vi "VI Linearisierung v2.vi"() -> ()   [LabVIEW 2020, in "Linearisierung v2.lvlib"] (continued)
      n463 = Select(t=T66."Disabled and Grayed Out" ("Deaktiviert"), s=w534, f=w533) -> (s? t:f=w550:T66)
      n464 = Select(t=FALSE ("x = y?"), s=w534, f=w552) -> (s? t:f=w554:T1)
      n465 = Select(t=u16 0, s=w534, f=w543) -> (s? t:f=w555:u16)
      n466 = Select(t=T66."Disabled and Grayed Out" ("Deaktiviert"), s=w535, f=w533) -> (s? t:f=w532:T66)
      n467 = property on="Gasteilerkorrektur" class="Bool."("Visible"=w534) -> (error out=w576:errorcluster)  [unwired: 2 in, 1 out]
      n468 = property on="Registerkarte" class="RKElem (strikt)"("Visible"=w574) -> (error out=w581:errorcluster)  [unwired: 2 in, 1 out]
      n469 = property on="Error" class="Cluster (strikt)"("Visible"=w574) -> (error out=w582:errorcluster)  [unwired: 2 in, 1 out]
      n470 = property on="Störung Kommunikation" class="Bool. (strikt)"("Visible"=w574) -> (error out=w583:errorcluster)  [unwired: 2 in, 1 out]
      n471 = property on="TCP Verbindung aktiv" class="Bool. (strikt)"("Visible"=w574) -> (error out=w584:errorcluster)  [unwired: 2 in, 1 out]
      n472 = property on="Error" class="Cluster (strikt)"("Visible"=w574) -> (error out=w578:errorcluster)  [unwired: 2 in, 1 out]
      n473 = property on="Anforderung" class="Bool. (strikt)"("Visible"=w574) -> (error out=w577:errorcluster)  [unwired: 2 in, 1 out]
      n474 = property on="ABBRECHEN" class="Bool."("Visible"=w574) -> (error out=w573:errorcluster)  [unwired: 2 in, 1 out]
      n475 = property on="STARTEN" class="Bool. (strikt)"("Visible"=w574) -> (error out=w572:errorcluster)  [unwired: 2 in, 1 out]
      n476 = property on="automatisch" class="Bool. (strikt)"("DisabledEnum"=w550, "Value"=w554) -> (error out=w558:errorcluster)  [unwired: 2 in, 1 out]
      n477 = property on="Gasteiler Span Eingänge" class="Ring (strikt)"("DisabledEnum"=w532, "Value"=w555, "Visible"=w519) -> (error out=w557:errorcluster)  [unwired: 2 in, 1 out]
      n478 = control-ref of="Eingabetabelle"() -> (w559:refnum<vi>)
      n479 = control-ref of="Ausgabetabelle"() -> (w542:refnum<vi>)
      n480 = control-ref of="EPA Ausgabetabelle"() -> (w563:refnum<vi>)
      n481 = control-ref of="LIN Ausgabetabelle"() -> (w562:refnum<vi>)
      n482 = local write "Gasteilerstatus"("" ("Gasteilerstatus")) -> ()
      n483 = call <vilib>:"Clear Errors.vi"("error in (no error)"=w596) -> ("error out"=w595:errorcluster)  [unwired: 5 in, 1 out]
      n484 = call "Einheiten finden.vi"("Komponente"=w568) -> ("Einheit in String"=w561:string)  [unwired: 6 in, 4 out]
      n485 = control-ref of="PDF single pages Components"() -> (w524:refnum<vi>)
      n486 = control-ref of="PDF single pages Span"() -> (w523:refnum<vi>)
      n487 = control-ref of="PDF Deckblatt"() -> (w522:refnum<vi>)
      n488 = control-ref of="PDF öffnen"() -> (w521:refnum<vi>)
      n489 = call "Einheiten in Tabellenspalten.vi"("Einheit"=w561, "Tabelle (Eingang)"=w559) -> ("Einheit out"=w560:string)  [unwired: 7 in, 2 out]
      n490 = local write "Einheit"(w561) -> ()
      n491 = local write "Einheit Deviation"(w561) -> ()
      n492 = call "Einheiten in Tabellenspalten.vi"("Einheit"=w560, "Tabelle (Eingang)"=w542) -> ("error out"=w567:errorcluster, "Einheit out"=w565:string)  [unwired: 7 in, 1 out]
      n493 = Bundle("PDF single pages Components"=w524, "PDF single pages Span"=w523, "PDF Deckblatt"=w522, "PDF öffnen"=w521) -> (w520:T130)  [unwired: 1 in]
      n494 = call "Einheiten in Tabellenspalten.vi"("error in (no error)"=w567, "Einheit"=w565, "Tabelle (Eingang)"=w563) -> ("error out"=w566:errorcluster, "Einheit out"=w564:string)  [unwired: 6 in, 1 out]
      n495 = Merge Errors(w576, w581, w582, w583, w584, w578, w577, w573, w572, w558, w557) -> (w580:errorcluster)
      n496 = call "GD_MG_MagicFormula_OnOff.vi"("Aktion"=enum16{"lesen", "schreiben", "init"}."init") -> ()  [unwired: 8 in, 2 out]
      n497 = call "Einheiten in Tabellenspalten.vi"("error in (no error)"=w566, "Einheit"=w564, "Tabelle (Eingang)"=w562) -> ()  [unwired: 6 in, 3 out]
      n498 = call <vilib>:"Clear Errors.vi"("error in (no error)"=w580) -> ()  [unwired: 5 in, 2 out]
    }
    frame #5 {
      # "#LIN_Hakerl"
      n499 = local read "TCP Verbindung aktiv"() -> (w668:bool)
      n500 = call "FGV CalGas.vi"("Aktionen"=FGV_CalGas_Aktionen."KAL extrahieren") -> ("Aufschaltung CalGas"=w650:T131)  [unwired: 6 in, 4 out]
      n501 = local write "Aufschaltung CalGas"(w650) -> ()
      n502 = Boolean To (0,1)(Boolean=w668) -> (0, 1=w667:i16)
      n503 = local write "Registerkarte"(w667) -> ()
      n504 = property on="FORTSETZEN" class="Bool."("Visible"=FALSE ("Sichtbar")) -> (error out=w653:errorcluster)  [unwired: 2 in, 1 out]
      n505 = call <vilib>:"Clear Errors.vi"("error in (no error)"=w653) -> ()  [unwired: 5 in, 2 out]
      n506 = call "Tabelle in die einzelnen Seiten zerlegen.vi"("Aktion"=FGV_Aktion_Tabelle_zerlegen."vereinzeln", "Index (Seite)"=41) -> ("Sprachliste"=w655:string[][])  [unwired: 7 in, 2 out]
      n507 = call "FGV Gasliste.vi"("Aktionen"=FGV_FT-IR_Gasliste_Aktionen."lesen") -> ("Aktuelle Gasliste gesamt"=w652:T48[])  [unwired: 8 in, 2 out]
      n508 = call "Tabelle in die einzelnen Seiten zerlegen.vi"("Aktion"=FGV_Aktion_Tabelle_zerlegen."vereinzeln", "Index (Seite)"=35) -> ("Sprachliste"=w661:string[][])  [unwired: 7 in, 2 out]
      n509 = call "Texte in VIs uebersetzen.vi"("Sprachliste"=w661, "String-Array zum Übersetzen"=w652, "String zum Übersetzen"="Temp. Messzelle" ("Neues Element/Teil-Array")) -> ("String-Array zum Übersetzen"=w659:string[], "String zum Übersetzen"=w663:string)  [unwired: 8 in, 3 out]
      n510 = call "String in Array suchen.vi"("Nach String/Zeichen suchen (-)"=w663, "String-Array"=w659) -> ("Index"=w665:i32)  [unwired: 7 in, 2 out]
      n511 = control-ref of="ABBRECHEN"() -> (w649:refnum<vi>)
      n512 = call "Texte in VIs uebersetzen.vi"("Sprachliste"=w655, "String zum Übersetzen"="Kalibrierung:" ("Status kalibrieren")) -> ("String zum Übersetzen"=w656:string)  [unwired: 9 in, 4 out]
      n513 = control-ref of="Ergebnis PDF TRUE"() -> (w643:refnum<vi>)
      n514 = control-ref of="Ergebnis PDF FALSE"() -> (w642:refnum<vi>)
      n515 = local write "Status kalibrieren"(w656) -> ()
      n516 = property class="Bool."(reference=w649, "DisabledEnum"=T66."Disabled and Grayed Out" ("Deaktiviert")) -> (reference out=w648:refnum<vi>, error out=w646:errorcluster)  [unwired: 1 in]
      n517 = Bundle By Name(cluster=T97 {"Yes Ctl Refnum"=refnum, "No Ctl Refnum"=refnum} ("ResultPictures"), "Yes Ctl Refnum"=w643, "No Ctl Refnum"=w642) -> (w641:T97)
      n518 = call <vilib>:"Clear Errors.vi"("error in (no error)"=w646) -> ()  [unwired: 5 in, 2 out]
      n519 = control-ref of="STARTEN"() -> (w645:refnum<vi>)
      "Ergebnis PDF TRUE" <- T3 TRUE ("Ergebnis PDF TRUE")
      "Ergebnis PDF FALSE" <- T3 FALSE ("Ergebnis PDF FALSE")
    }
    frame #6 {
      # "War der GD ein Horiba GDC und das VI wurde\ngestoppt, stimmen beim Start die Error Flags nicht ...."
      n520 = local read "Gasteiler Type"() -> (w671:T15)
      n521 = property on="Gasteiler Type" class="Ring (strikt)"("Val(Sgnl)"=w671) -> (error out=w670:errorcluster)  [unwired: 2 in, 1 out]
      n522 = call <vilib>:"Clear Errors.vi"("error in (no error)"=w670) -> ()  [unwired: 5 in, 2 out]
    }
    frame #7 {
      n523 = Wait Until Next ms Multiple(millisecond multiple=u32 200 ("ms")) -> (millisecond timer value=w672:u32)
      n524 = flat-sequence {
        tunnel: w672 -> [_]
        frame #0 {
          n525 = call "Spantabellenanzeige.vi"() -> ("SpanTabelle"=w676:T48[][])  [unwired: 10 in, 1 out]
          n526 = Delete From Array(array=w676, length=3 ("Länge"), index (col)=0 ("Deaktivierter Index (Spalte)")) -> (deleted portion=→"SpanTabelleAnzeige":T48[][], array with subset deleted=w677:T48[][])  [unwired: 1 in]
          n527 = local write "SpanTabelleEingabe"(w677) -> ()
        }
      }
    }
    frame #8 {
      w683 = T4 FALSE  # Gasteiler Spülen
      n528 = call "FT-IR EVID-Codes External Data.vi"("Aktionen"=Aktionen_EVID-Codes."lesen") -> ("Anzahl"=w698:i32)  [unwired: 9 in, 5 out]
      n529 = call "FGV Gasliste.vi"("Aktionen"=FGV_FT-IR_Gasliste_Aktionen."lesen") -> ("Aktuelle Gasliste gesamt"=w689:T48[], "Aktuelle Gasliste FT-IR"=w696:T48[])  [unwired: 8 in, 1 out]
      n530 = call "FGV Span.vi"("Aktion"=Aktion_FGV_Span."Seite aktiv", "Aktiv"=FALSE) -> ()  [unwired: 6 in, 4 out]
      n531 = Add(x=w698, y=3) -> (x+y=w688:i32)
      n532 = control-ref of="SpanTabelleEingabe"() -> (w681:refnum<vi>)
      n533 = Array Size(array=w696) -> (size(s)=w695:i32)
      n534 = Array Size(array=w689) -> (size(s)=w690:i32)
      n535 = control-ref of="PolynomTabelleAnzeige"() -> (w679:refnum<vi>)
      n536 = control-ref of="PolynomTabelleEingabe"() -> (w680:refnum<vi>)
      n537 = disable-structure shown="Deaktiviert" {
        disable-tunnel: w680 -> [w703 _]
        frame Disabled {
          n538 = for {
            N: 5 -> [_]
            tunnel: w703 -> [w707]
            tunnel: T100 {"Row"=0, "Column"=0} ("Aktive Zelle:Aktive Zelle") -> [w706]
            i -> [w705]
            n539 = for {
              N: 200 -> [_]
              tunnel: w707 -> [w714]
              tunnel: w706 -> [w713]
              tunnel: w705 -> [w711]
              i -> [w710]
              n540 = Bundle By Name(cluster=w713, "Column"=w711, "Row"=w710) -> (w712:T100)
              n541 = property class="Tbl (strikt)"(reference=w714, "Active Cell"=w712) -> (reference out=w709:refnum<vi>)  [unwired: 1 in, 1 out]
              n542 = property class="Tbl (strikt)"(reference=w709, "Justify"=enum16{"Left", "Center", "Right"}."Left" ("Aktive Zelle:Zellenausrichtung")) -> ()  [unwired: 1 in, 2 out]
            }
          }
        }
        frame Enabled {
        }
      }
      n543 = Subtract(x=w695, y=w688) -> (x-y=w694:i32)
      n544 = Subtract(x=w690, y=w688) -> (x-y=w687:i32)
      n545 = control-ref of="SpanTabelleAnzeige"() -> (w682:refnum<vi>)
      n546 = call "Zeile faerben.vi"("Anzahl"=w694, "Table (Eingang)"=w682) -> ("error out"=w693:errorcluster)  [unwired: 9 in]
      n547 = call "Zeile faerben.vi"("error in (no error)"=w693, "Anzahl"=w694, "Table (Eingang)"=w681) -> ("error out"=w692:errorcluster)  [unwired: 8 in]
      n548 = call "Zeile faerben.vi"("error in (no error)"=w692, "Anzahl"=w687, "Table (Eingang)"=w680) -> ("error out"=w691:errorcluster)  [unwired: 8 in]
      n549 = call "Zeile faerben.vi"("error in (no error)"=w691, "Anzahl"=w687, "Table (Eingang)"=w679) -> ()  [unwired: 8 in, 1 out]
      n550 = disable-structure shown="TestRun==TRUE" {
        disable-tunnel: [w715 w716] -> w684
        frame condition #0 (active) {
          w715 = TRUE  # TestRun
          # "#TestRun"
        }
        frame condition #1 {
          w716 = FALSE  # TestRun
        }
      }
    }
  }
  n551 = while {
    tunnel: w39 -> [w760]
    tunnel: w37 -> [_]
    shift-right: [w758] -> _
    shift-left: w17 -> [w757]
    shift-right: [w756] -> _
    shift-left: _ -> [w755]
    shift-right: [w754] -> _
    shift-left: _ -> [w753]
    tunnel: w36 -> [w752]
    tunnel: w35 -> [w751]
    tunnel: w34 -> [w750]
    tunnel: w33 -> [w749]
    tunnel: w32 -> [w748]
    tunnel: w31 -> [w747]
    tunnel: w30 -> [w746]
    tunnel: w29 -> [w745]
    tunnel: w28 -> [w744]
    tunnel: w25 -> [w743]
    tunnel: w26 -> [w742]
    tunnel: w27 -> [w741]
    tunnel: w24 -> [w740]
    tunnel: w23 -> [w739]
    tunnel: w19 -> [w738]
    tunnel: w20 -> [w737]
    tunnel: w21 -> [w736]
    tunnel: w22 -> [w735]
    tunnel: w18 -> [w734]
    tunnel: w16 -> [w733]
    tunnel: w15 -> [w732]
    tunnel: w14 -> [w731]
    tunnel: w13 -> [w730]
    tunnel: w12 -> [w729]
    shift-right: [w728] -> _
    shift-left: w38 -> [w759]
    tunnel: w11 -> [w727]
    tunnel: w10 -> [w726]
    tunnel: w9 -> [w725]
    tunnel: w8 -> [w724]
    tunnel: w7 -> [w723]
    tunnel: w6 -> [w722]
    tunnel: w5 -> [w721]
    tunnel: w4 -> [w720]
    tunnel: w3 -> [w718]
    tunnel: w2 -> [w719]
    tunnel: w1 -> [w717]
    stop <- FALSE stop-if-true
    # "250 für Timer"
    n552 = event shown="[26] \"EPA PDF erzeugen\": Wertänderung" {
      selector: _ -> [_ _ _ _ _ _ _ _ _ _ _ _ _ _ _ _ _ _ _ _ _ _ _ _ _ _ _ _ _ _ _ _ _ _ _ _ _ _ _ _ _ _ _ _ _ _ _ _ _ _ _ _ _ _ _ _ _ _ _ _ _]
      dyn-events: _ -> [_ _ _ _ _ _ _ _ _ _ _ _ _ _ _ _ _ _ _ _ _ _ _ _ _ _ _ _ _ _ _ _ _ _ _ _ _ _ _ _ _ _ _ _ _ _ _ _ _ _ _ _ _ _ _ _ _ _ _ _ _]
      timeout: 250 -> [_ _ _ _ _ _ _ _ _ _ _ _ _ _ _ _ _ _ _ _ _ _ _ _ _ _ _ _ _ _ _ _ _ _ _ _ _ _ _ _ _ _ _ _ _ _ _ _ _ _ _ _ _ _ _ _ _ _ _ _ _]
      tunnel: w760 -> [w768 _ _ _ _ _ _ _ _ _ _ _ _ _ _ w1488 w1532 w1567 _ _ w1742 w1765 w1809 _ _ w2079 w2473 _ _ _ _ _ w2652 _ w2893 w2999 w3024 _ w3060 _ _ _ w3174 _ w3242 _ _ _ _ _ _ _ _ _ _ _ _ _ _ _ _]
      tunnel: w759 -> [w796 w1237 w1243 _ w1316 w1333 w1360 w1372 w1388 w1400 w1412 w1430 w1442 w1446 w1459 w1485 w1514 w1565 w1717 w1722 w1739 w1762 w1806 w1844 w1863 w2064 w2479 w2505 w2514 w2521 w2580 w2605 w2628 w2842 w2892 w3000 w3023 w3043 w3057 w3120 w3128 w3148 w3179 w3210 w3244 w3481 w3574 w3584 w3620 w3759 w3812 w3848 w3864 w3888 w4033 w4111 w4115 w4140 w4180 w4341 w4372]
      tunnel: [w810 w1239 w1245 w1278 w1325 w1339 w1364 w1380 w1392 w1404 w1421 w1434 w1445 w1458 w1467 w1491 w1533 w1573 w1721 w1724 w1741 w1764 w1808 w1850 w1872 w2086 w2481 w2507 w2516 w2535 w2587 w2609 w2653 w2857 w2896 w3002 w3033 w3046 w3059 w3127 w3134 w3150 w3198 w3220 w3253 w3494 w3579 w3590 w3650 w3785 w3841 w3863 w3872 w3932 w4080 w4114 w4121 w4143 w4231 w4356 w4374] -> w758
      tunnel: w757 -> [w811 w1239 w1245 w1278 w1325 w1339 w1364 w1380 w1392 w1404 w1421 w1434 w1445 w1458 w1467 w1491 w1533 w1573 w1721 _ w1741 w1764 w1808 w1850 w1872 w2086 w2481 w2507 w2516 w2535 w2587 w2609 w2653 w2857 w2896 w3002 w3033 w3046 w3059 w3127 w3134 w3150 w3198 w3220 w3253 w3494 w3579 w3590 w3650 w3785 w3841 w3863 w3872 w3932 w4080 w4114 w4121 w4143 w4231 w4356 w4374]
      tunnel: [w807 w1238 w1244 w1277 w1324 w1338 w1363 w1379 w1391 w1403 w1420 w1433 w1444 w1457 w1466 w1486 w1531 w1566 w1718 w1723 w1740 w1763 w1807 w1846 w1871 w2085 w2480 w2506 w2515 w2534 w2583 w2608 w2649 w2846 w2895 w3001 w3032 w3045 w3058 w3125 w3133 w3149 w3197 w3219 w3251 w3493 w3578 w3589 w3649 w3784 w3840 w3862 w3871 w3928 w4079 w4112 w4120 w4142 w4230 w4355 w4373] -> w756
      tunnel: w755 -> [w808 w1238 w1244 w1277 w1324 w1338 w1363 w1379 w1391 w1403 w1420 w1433 w1444 w1457 w1466 w1486 w1531 w1566 w1718 w1723 w1740 w1763 w1807 w1846 w1871 w2085 w2480 w2506 w2515 w2534 w2583 w2608 w2649 w2846 w2895 w3001 w3032 w3045 w3058 w3125 w3133 w3149 w3197 w3219 w3251 w3493 w3578 w3589 w3649 w3784 w3840 w3862 w3871 w3928 w4079 w4112 w4120 w4142 w4230 w4355 w4373]
      tunnel: [w806 _ _ _ _ _ _ _ _ _ _ _ _ _ _ _ _ _ _ _ _ _ _ _ _ _ _ _ _ _ _ _ _ _ _ _ _ _ _ _ _ _ _ _ _ _ _ _ _ _ _ _ _ _ _ _ _ _ _ _ _] -> w754
      tunnel: w753 -> [w805 _ _ _ _ _ _ _ _ _ _ _ _ _ _ _ _ _ _ _ _ _ _ _ _ _ _ _ _ _ _ _ _ _ _ _ _ _ _ _ _ _ _ _ _ _ _ _ _ _ _ _ _ _ _ _ _ _ _ _ _]
      tunnel: w752 -> [_ _ _ _ w1323 w1337 w1361 w1378 w1389 w1401 w1419 w1431 _ _ _ _ _ _ _ _ _ _ _ _ _ _ _ _ _ _ _ _ _ _ _ _ _ _ _ _ _ _ _ _ _ _ _ _ _ _ _ _ _ _ _ _ _ _ _ _ _]
      tunnel: w751 -> [_ _ _ _ _ _ _ _ _ _ _ _ _ _ _ _ _ _ _ _ _ _ _ _ _ _ _ _ _ _ _ _ _ _ _ _ _ _ _ _ _ _ _ _ _ _ _ _ _ _ _ _ _ _ w4065 _ _ _ _ _ _]
      tunnel: w750 -> [_ _ _ _ _ _ _ _ _ _ _ _ _ _ _ _ _ _ _ _ _ _ _ _ _ _ _ _ _ _ _ _ w2638 _ _ _ _ _ _ _ _ _ w3190 _ w3238 w3484 _ _ _ _ _ _ _ w3899 _ _ _ _ _ _ _]
      tunnel: w749 -> [_ _ _ _ _ _ _ _ _ _ _ _ _ _ _ _ _ _ _ _ _ _ _ _ _ _ _ _ _ _ _ _ w2635 _ _ _ _ _ _ _ _ _ w3187 _ w3233 _ _ _ _ _ _ _ _ _ _ _ _ _ _ _ _]
      tunnel: w748 -> [_ _ _ _ _ _ _ _ _ _ _ _ _ _ _ _ _ _ _ _ _ _ _ _ _ _ _ _ _ _ _ _ _ _ _ _ _ _ _ _ _ _ w3196 _ _ _ _ _ _ _ _ _ _ _ _ _ _ _ _ _ _]
      tunnel: w747 -> [_ _ _ _ _ _ _ _ _ _ _ _ _ _ _ _ _ _ _ _ _ _ _ _ _ _ _ _ _ _ _ _ w2637 _ _ _ _ _ _ _ _ _ w3189 _ w3235 _ _ _ _ _ _ _ _ _ _ _ _ _ _ _ _]
      tunnel: w746 -> [_ _ _ _ _ _ _ _ _ _ _ _ _ _ _ _ _ _ _ _ _ _ _ _ _ _ _ _ _ _ _ _ w2636 _ _ _ _ _ _ _ _ _ w3188 _ w3234 w3489 _ _ _ _ _ _ _ w3902 _ _ _ _ _ _ _]
      tunnel: w745 -> [w775 _ _ _ _ _ _ _ _ _ _ _ _ _ _ _ _ _ _ _ _ _ _ _ _ w2078 w2478 _ _ _ _ _ w2645 w2843 _ _ _ _ _ w3122 _ _ _ _ _ _ _ _ _ _ _ _ _ _ _ _ _ _ _ _ _]
      tunnel: w744 -> [w782 _ _ _ _ _ _ _ _ _ _ _ _ _ _ _ _ _ _ _ _ _ _ _ _ _ _ _ _ _ _ _ w2642 _ _ _ _ _ _ _ _ _ _ _ _ _ _ _ _ _ _ _ _ _ _ _ _ _ _ _ _]
      tunnel: w743 -> [_ _ _ _ _ _ _ _ _ _ _ _ _ _ _ _ _ _ _ _ _ _ _ _ w1868 _ _ _ _ _ _ _ w2632 _ _ _ _ _ _ _ _ _ w3185 _ w3229 w3452 _ _ w3646 _ _ w3849 _ _ _ _ _ _ _ _ _]
      tunnel: w742 -> [_ _ _ _ _ _ _ _ _ _ _ _ _ _ _ _ _ _ _ _ _ _ _ _ w1866 _ _ _ _ _ _ _ _ _ _ _ _ _ _ _ _ _ _ _ _ _ _ _ w3644 _ _ _ _ _ _ _ _ _ _ _ _]
      tunnel: w741 -> [_ _ _ _ _ _ _ _ _ _ _ _ _ _ _ _ _ _ _ _ _ _ _ _ w1867 _ _ _ _ _ _ _ _ _ _ _ _ _ _ _ _ _ _ _ _ _ _ _ w3645 _ _ _ _ _ _ _ _ _ _ _ _]
      tunnel: w740 -> [_ _ _ _ _ _ _ _ _ _ _ _ _ _ _ _ _ _ _ _ _ _ _ _ _ _ _ _ _ _ _ _ w2634 _ _ _ _ _ _ _ _ _ w3186 _ w3230 w3453 _ _ w3643 _ _ w3850 _ _ _ _ _ _ _ _ _]
      tunnel: w739 -> [_ _ _ _ _ _ _ _ _ _ _ _ _ _ _ _ _ _ _ _ _ _ _ _ _ _ _ _ _ _ _ _ _ _ _ _ _ _ _ _ _ _ _ _ _ _ _ _ _ _ _ _ _ _ w4034 _ _ _ _ _ _]
      tunnel: w738 -> [_ _ _ _ _ _ _ _ _ _ _ _ _ _ _ _ _ _ _ _ _ _ _ _ _ _ _ _ _ _ _ _ _ _ _ _ _ _ _ _ _ _ _ _ _ _ _ _ _ _ _ _ _ _ _ _ _ _ w4192 _ _]
      tunnel: w737 -> [_ _ _ _ _ _ _ _ _ _ _ _ _ _ _ _ _ _ _ _ _ _ _ _ _ _ _ _ _ _ _ _ _ _ _ _ _ _ _ _ _ _ _ _ _ _ _ _ _ _ _ _ _ _ _ _ _ _ w4191 _ _]
      tunnel: w736 -> [w798 _ _ _ _ _ _ _ _ _ _ _ _ _ _ _ _ _ _ _ _ _ _ _ w1861 _ _ _ _ _ _ _ _ _ _ _ _ _ _ _ _ _ _ _ _ _ _ _ _ _ _ _ _ _ _ _ _ _ w4184 w4348 _]
      tunnel: w735 -> [w797 _ _ _ _ _ _ _ _ _ _ _ _ _ _ _ _ _ _ _ _ _ _ _ w1862 _ _ _ _ _ _ _ _ _ _ _ _ _ _ _ _ _ _ _ _ _ _ _ _ _ _ _ _ _ _ _ _ _ w4183 w4347 _]
      tunnel: w734 -> [_ _ _ _ _ _ _ _ _ _ _ _ _ _ _ _ _ _ _ _ _ _ _ _ _ _ _ _ _ _ _ _ w2627 _ _ _ _ _ _ _ _ _ w3171 _ w3231 _ _ _ _ _ _ _ w3870 _ _ _ _ _ _ _ _]
      tunnel: w733 -> [w776 _ _ _ _ _ _ _ _ _ _ _ _ _ _ _ _ _ _ _ _ _ _ _ _ _ _ _ _ _ _ _ _ _ _ _ _ _ _ _ _ _ _ _ _ _ _ _ _ _ _ _ _ _ _ _ _ _ _ _ _]
      tunnel: w732 -> [_ _ _ w1276 _ _ _ _ _ _ _ _ _ _ _ _ _ _ _ _ _ _ _ _ _ _ _ _ _ _ _ _ _ _ _ _ _ _ _ _ _ _ _ _ _ _ _ _ _ _ _ _ _ _ _ _ _ _ _ _ _]
      tunnel: w731 -> [_ _ _ w1275 _ _ _ _ _ _ _ _ _ _ _ _ _ _ _ _ _ _ _ _ _ _ _ _ _ _ _ _ _ _ _ _ _ _ _ _ _ _ _ _ _ _ _ _ _ _ _ _ _ _ _ _ _ _ _ _ _]
      tunnel: w730 -> [_ _ _ w1274 _ _ _ _ _ _ _ _ _ _ _ _ _ _ _ _ _ _ _ _ _ _ _ _ _ _ _ _ _ _ _ _ _ _ _ _ _ _ _ _ _ _ _ _ _ _ _ _ _ _ _ _ _ _ _ _ _]
      tunnel: w729 -> [_ _ _ w1273 _ _ _ _ _ _ _ _ _ _ _ _ _ _ _ _ _ _ _ _ _ _ _ _ _ _ _ _ _ _ _ _ _ _ _ _ _ _ _ _ _ _ _ _ _ _ _ _ _ _ _ _ _ _ _ _ _]
      tunnel: [w796 w1237 w1243 w1272 w1316 w1333 w1360 w1372 w1388 w1400 w1412 w1430 w1442 w1446 w1459 w1485 w1514 w1565 w1717 w1722 w1739 w1762 w1806 w1844 w1863 w2064 w2479 w2505 w2514 w2521 w2580 w2605 w2628 w2842 w2892 w3000 w3023 w3043 w3057 w3120 w3128 w3148 w3179 w3210 w3244 w3481 w3574 w3584 w3620 w3759 w3812 w3848 w3864 w3888 w4033 w4111 w4115 w4140 w4180 w4341 w4372] -> w728
      tunnel: w727 -> [_ _ w1242 _ _ _ _ _ _ _ _ _ _ _ _ _ _ _ _ _ _ _ _ _ _ _ _ _ _ _ _ _ _ _ _ _ _ _ _ _ _ _ _ _ _ _ _ _ _ _ _ _ _ _ _ _ _ _ _ _ _]
      tunnel: w726 -> [_ _ w1241 _ _ _ _ _ _ _ _ _ _ _ _ _ _ _ _ _ _ _ _ _ _ _ _ _ _ _ _ _ _ _ _ _ _ _ _ _ _ _ _ _ _ _ _ _ _ _ _ _ _ _ _ _ _ _ _ _ _]
      tunnel: w725 -> [_ _ w1240 _ _ _ _ _ _ _ _ _ _ _ _ _ _ _ _ _ _ _ _ _ _ _ _ _ _ _ _ _ _ _ _ _ _ _ _ _ _ _ _ _ _ _ _ _ _ _ _ _ _ _ _ _ _ _ _ _ _]
      tunnel: w724 -> [_ _ _ _ _ _ _ _ _ _ _ _ _ _ _ _ _ _ _ _ _ _ _ _ _ w2059 _ _ _ _ _ _ _ _ _ _ _ _ _ _ _ _ _ _ _ _ _ _ _ _ _ _ _ _ _ _ _ _ _ _ _]
      tunnel: w723 -> [_ _ _ _ _ _ _ _ _ _ _ _ _ _ _ _ _ _ _ _ _ _ _ _ _ w2056 w2475 _ _ _ _ _ _ _ _ _ _ _ _ _ _ _ _ _ _ _ _ _ _ _ _ _ _ _ _ _ _ _ _ _ _]
      tunnel: w722 -> [_ _ _ _ _ _ _ _ _ _ _ _ _ _ _ _ _ _ _ _ _ _ _ _ _ w2055 w2476 _ _ _ _ _ _ _ _ _ _ _ _ _ _ _ _ _ _ _ _ _ _ _ _ _ _ _ _ _ _ _ _ _ _]
      tunnel: w721 -> [_ _ _ _ _ _ _ _ _ _ _ _ _ _ _ _ _ _ _ _ _ _ _ _ _ w2054 w2477 _ _ _ _ _ _ _ _ _ _ _ _ _ _ _ _ _ _ _ _ _ _ _ _ _ _ _ _ _ _ _ _ _ _]
      tunnel: w720 -> [_ _ _ _ _ _ _ _ _ _ _ _ _ _ _ _ _ _ _ _ _ _ _ _ _ w2049 w2474 _ _ _ _ _ _ _ _ _ _ _ _ _ _ _ _ _ _ _ _ _ _ _ _ _ _ _ _ _ _ _ _ _ _]
      tunnel: w718 -> [_ _ _ _ _ _ _ _ _ _ _ _ _ _ _ _ _ _ _ _ _ _ _ _ _ w2047 _ w2499 _ _ _ _ _ _ _ _ _ _ _ _ _ _ _ _ _ _ _ _ w3611 _ _ _ _ _ _ _ _ _ _ _ _]
      tunnel: w719 -> [_ _ _ _ _ _ _ _ _ _ _ _ _ _ _ _ _ _ _ _ _ _ _ _ _ _ _ _ _ _ _ _ _ _ _ _ _ _ _ _ _ _ w3168 _ w3227 w3436 _ _ _ _ _ _ _ _ _ _ _ _ _ _ _]
      tunnel: w717 -> [_ _ _ _ _ _ _ _ _ _ _ _ _ _ _ _ _ _ _ _ _ _ _ _ _ _ _ w2500 w2513 _ _ _ _ _ _ _ _ _ _ _ _ _ _ _ _ _ _ _ w3610 _ _ _ _ _ _ _ _ _ _ _ _]
      event Timeout {
        w769 = TRUE  # get Test Data
        n553 = event-data() -> ("Source"=w784:T158, "Type"=w786:T159, "Time"=w785:u32)  [unwired: 1 in]
        n554 = control-ref of="FORTSETZEN"() -> (w774:refnum<vi>)
        n555 = control-ref of="Speichern LIN"() -> (w773:refnum<vi>)
        n556 = call "GD_MG_MagicFormula_OnOff.vi"("Aktion"=enum16{"lesen", "schreiben", "init"}."lesen") -> ("use old LNI"=w787:bool, "MG_use_magic_formula"=w788:bool)  [unwired: 8 in]
        n557 = local read "Hauptregisterkarte"() -> (w813:T8)
        n558 = call "Komponentenausgabe.vi"() -> ("Gaskomponente"=w814:T7)  [unwired: 8 in, 3 out]
        n559 = call "FGV Daten Abholung uebergeben.vi"("Aktion"=Aktion_FGV_Daten_Abholung_uebergebenctl."lesen") -> ("Zustand"=w803:string, "Anzeige aktualisieren"=w802:bool, "Beendet"=w781:bool, "Restlaufzeit out"=w799:sgl)  [unwired: 10 in, 1 out]
        n560 = call "Editierte Zelle merken.vi"("Aktion"=enum16{"init", "lesen", "schreiben"}."schreiben") -> ()  [unwired: 9 in, 2 out]
        n561 = call "FGV Stoerungen sammeln und auswerten.vi"("Aktion"=Aktion_FGV_Stoerungen_sammeln_und_auswerten."prüfen") -> ("Error"=w770:bool)  [unwired: 12 in, 6 out]
        n562 = local write "MG_use_magic_formula"(w788) -> ()
        n563 = local write "use old LNI"(w787) -> ()
        n564 = Bundle By Name(cluster=T135 {"STARTEN"=refnum, "Abbrechen (Eingang)"=refnum, "FORTSETZEN"=refnum, "Speichern LIN"=refnum} ("Referenzen Cluster"), "STARTEN"=w776, "Abbrechen (Eingang)"=w775, "FORTSETZEN"=w774, "Speichern LIN"=w773) -> (w771:T135)
        n565 = case shown="\"HovaCAL Interface\"" w813 {
          tunnel: w814 -> [_ _ w915 w954 _ _ w1135 w1161 _ _]
          tunnel: w811 -> [w895 w907 w912 w962 w1013 w1089 w1138 w1160 w1176 w1214]
          tunnel: [w895 w907 w912 w962 w1012 w1089 w1138 w1160 w1176 w1214] -> w810
          tunnel: w808 -> [w894 w906 w911 w961 w1008 w1088 w1137 w1159 w1171 w1213]
          tunnel: [w894 w906 w911 w961 w1008 w1088 w1137 w1159 w1168 w1213] -> w807
          tunnel: [w893 w905 w910 w960 w1007 w1087 w1136 w1158 w1169 w1201] -> w806
          tunnel: w805 -> [w893 w905 w910 w960 w1007 w1087 w1136 w1158 w1169 w1212]
          tunnel: w803 -> [_ _ _ _ _ w1071 _ _ _ _]
          tunnel: w802 -> [_ _ _ _ _ w1086 _ _ _ _]
          tunnel: w781 -> [_ _ _ _ _ w1085 _ _ _ _]
          tunnel: w798 -> [_ w904 _ _ _ _ _ _ _ _]
          tunnel: w799 -> [_ _ _ _ _ w1083 _ _ _ _]
          tunnel: w797 -> [_ w903 _ _ _ _ _ _ _ _]
          tunnel: w786 -> [_ _ _ _ _ _ _ _ _ _]
          tunnel: w785 -> [_ _ _ _ _ _ _ _ _ _]
          tunnel: w784 -> [_ _ _ _ _ _ _ _ _ _]
          tunnel: w768 -> [_ _ _ _ _ w1072 _ _ _ _]
          tunnel: w769 -> [_ _ _ _ _ w1069 _ _ _ _]
          frame "Einstellungen", Default {
            # "wird auch wo andes gesetzt (HovaCAL Interference Test)\n#HovaCAL_Interference_BugFixes"
            # "#MG_GK_back_calc"
            n566 = call "FGV Passwortlevel.vi"("FGV Passwort Aktion"=FGV_Passwort_Aktion."lesen") -> ("aktueller Level"=w891:i16)  [unwired: 8 in, 2 out]
            n567 = call "FGV cRIO-Daten.vi"("Aktion"=enum16{"lesen", "schreiben"}."lesen") -> ("Analog Input"=w896:T160)  [unwired: 9 in, 9 out]
            n568 = disable-structure shown="OFS==FALSE, Standard" {
              disable-tunnel: [w900 w902] -> w897
              disable-tunnel: w896 -> [w899 w901]
              frame condition #0 (active) {
                # "AI4: Druck CalGas"
                n569 = Unbundle By Name(w899) -> ("AI4: Druck CalGas"=w900:sgl)
              }
              frame condition #1 {
                # "AI4: Druck FT-IR Messzelle"
                n570 = Unbundle By Name(w901) -> ("AI4: Druck CalGas"=w902:sgl)
              }
            }
            "Druck CG zu Gasteiler:" <- w897
            n571 = Greater?(x=w891, y=i16 9) -> (0:w892:bool)
            n572 = property on="use old LNI" class="Bool. (strikt)"("Visible"=w892) -> (error out=w888:errorcluster)  [unwired: 2 in, 1 out]
            n573 = property on="MG_use_magic_formula" class="Bool. (strikt)"("Visible"=w892) -> (error out=w889:errorcluster)  [unwired: 2 in, 1 out]
            n574 = Merge Errors(w888, w889) -> (w890:errorcluster)
            n575 = call <vilib>:"Clear Errors.vi"("error in (no error)"=w890) -> ()  [unwired: 5 in, 2 out]
            n576 = call "FGV Gasteiler.vi"("Aktionen"=Aktionen_FGV_Gasteiler_Daten."lesen") -> ("Anforderung"=w884:bool)  [unwired: 11 in, 7 out]
            n577 = local write "Anforderung"(w884) -> ()
          }
          frame "Span Einstellungen" {
            n578 = disable-structure shown="Deaktiviert" {
              disable-tunnel: w904 -> [w909 _]
              disable-tunnel: w903 -> [w908 _]
              frame Disabled {
                # "hier nicht !!!"
                n579 = call "Span Register setzen.vi"("GD Span Eingänge"=w908, "automatisch Boolesch (Eingang)"=w909) -> ()  [unwired: 3 in, 7 out]
              }
              frame Enabled {
              }
            }
          }
          frame "HovaCal Einstellungen" {
            n580 = call "FGV Gasliste.vi"("Aktionen"=FGV_FT-IR_Gasliste_Aktionen."lesen") -> ("Aktuelle Gasliste gesamt"=w920:T48[])  [unwired: 8 in, 2 out]
            n581 = Build Array (concatenate)("----", w920) -> (w918:T48[])
            n582 = Increment(x=w915) -> (x+1=w917:T7)
            n583 = Index Array(array=w918, index=w917) -> (element=→"Komponente HovaCal":T48)
            n584 = call "FGV_Betreibsdaten.vi"("Enum"=Aktion_FGV_Betriebsdaten."Lesen" ("Aktion")) -> ("Dynamische Werte 2"=→"Dynamische Werte":T62)  [unwired: 11 in, 7 out]
          }
          frame "HovaCAL Interface" {
            # "#HovaCALInterface"
            n585 = call "FGV_HovaCAL_Interface_GetData.vi"("Aktion"=Aktion_FGV_HovaCAL_Interface_GetData."lesen") -> ("first flags out"=w946:T151)  [unwired: 6 in, 4 out]
            n586 = call "FGV_HovaCAL_Interface_Kommandos.vi"("Aktion"=Aktion_FGV_HovaCAL_Interface_Kommandos."lesen") -> ("gesammelt ?"=w933:bool)  [unwired: 4 in, 5 out]
            n587 = Unbundle By Name(w946) -> ("first contact in"=w941:bool, "first actual values in"=w945:bool)
            n588 = property on="HovaCALInterface-Freigabe" class="Bool."("Visible"=w933) -> (error out=w949:errorcluster)  [unwired: 2 in, 1 out]
            n589 = Not(x=w933) -> (.not. x?=w931:bool)
            n590 = call "FGV Gasliste.vi"("Aktionen"=FGV_FT-IR_Gasliste_Aktionen."lesen") -> ("Aktuelle Gasliste gesamt"=w958:T48[])  [unwired: 8 in, 2 out]
            n591 = call <vilib>:"Clear Errors.vi"("error in (no error)"=w949) -> ()  [unwired: 5 in, 2 out]
            n592 = Build Array (concatenate)("----", w958) -> (w956:T48[])
            n593 = Increment(x=w954) -> (x+1=w955:T7)
            n594 = call "Verzoegerung PC.vi"("sec"=u16 1, "Startsignal"=w945) -> ("Zeit abgelaufen?"=w942:bool)  [unwired: 8 in, 1 out]
            n595 = call "Verzoegerung PC.vi"("sec"=u16 1, "Startsignal"=w931) -> ("Zeit abgelaufen?"=w930:bool)  [unwired: 8 in, 1 out]
            n596 = Index Array(array=w956, index=w955) -> (element=→"Komponente HovaCal Interface":T48)
            n597 = And(x=w942, y=w930) -> (x .and. y?=w932:bool)
            n598 = case shown="True" w932 {
              tunnel: w941 -> [_ _]
              tunnel: [_ w975] -> w947
              frame False {
              }
              frame True {
                # "#HovaCAL_Interference_BugFixes"
                n599 = disable-structure shown="TestRun==TRUE" {
                  disable-tunnel: [w993 w1000] -> w981
                  disable-tunnel: [w992 w999] -> w980
                  disable-tunnel: [w991 _] -> w979
                  disable-tunnel: [w990 w1001] -> w978
                  disable-tunnel: [w989 w997] -> w977
                  disable-tunnel: [w988 w995] -> w976
                  disable-tunnel: [w987 _] -> w975
                  disable-tunnel: [w986 w1002] -> w974
                  disable-tunnel: [w985 w998] -> w968
                  frame condition #0 {
                    n600 = call "Set Values From HovaCAL Input.vi"() -> ("error out"=w987:errorcluster, "HovaCAL Temperature"=w989:dbl[], "SetPumpMode-Cluster"=w990:T163, "Cluster.PumpModeGeneral"=w992:T166, "Pump Concentrations-Cluster"=w985:T167[], "Set Values Cluster"=w986:T168, "Flow Input Cluster"=w988:cluster{"total flow setpoint":dbl}, "Limits Cluster"=w993:cluster{"flow":dbl[], "temp":dbl[]}, "SetPumpMode"=w991:cluster{"run":bool})  [unwired: 3 in]
                  }
                  frame condition #1 (active) {
                    # "#HovaCAL_Interference_BugFixes"
                    n601 = call "FGV_HovaCAL_Interface_SetData.vi"("Aktion"=Aktion_FGV_HovaCAL_Interface_SetData."lesen") -> ("PumpModeGeneral-Cluster out"=w999:T166, "Set Values Cluster out"=w1002:T168, "PumpMode-Cluster out"=w1001:T169, "total flow setpoint out"=w994:dbl, "Temperature out"=w997:dbl[], "Limits Cluster out"=w1000:cluster{"flow":dbl[], "temp":dbl[]}, "Pump Concentrations-Cluster out"=w998:T167[])  [unwired: 8 in]
                    n602 = Bundle By Name(cluster=cluster{"total flow setpoint":dbl} {"total flow setpoint"=0.0} ("Flow Input Cluster"), "total flow setpoint"=w994) -> (w995:cluster{"total flow setpoint":dbl})
                  }
                }
                n603 = call <vilib>:"Clear Errors.vi"("error in (no error)"=w975) -> ()  [unwired: 5 in, 2 out]
                n604 = local write "HovaCAL SetPumpMode"(w979) -> ()
                n605 = local write "HovaCAL Cluster.PumpModeGeneral"(w980) -> ()
                n606 = local write "HovaCAL SetPumpMode-Cluster"(w978) -> ()
                n607 = local write "HovaCAL Limits Cluster"(w981) -> ()
                n608 = local write "HovaCAL Flow Input Cluster"(w976) -> ()
                n609 = local write "HovaCAL Temperature"(w977) -> ()
                n610 = Index Array(array=w968) -> (element #1=w966:T167, element #2=w965:T167)  [unwired: 2 in]
                n611 = Index Array(array=w974) -> (element #1=w973:T170, element #2=w972:T170, element #3=w971:T170, element #4=w970:T170, element #5=w969:T170)  [unwired: 5 in]
                n612 = call "Pump Concentrations in Procent.vi"("Pump Concetrations-Cluster (Eingang)"=w966) -> ("Pump Concetrations-Cluster (Ausgang)"=w967:T167)  [unwired: 10 in]
                n613 = call "Pump Concentrations in Procent.vi"("Pump Concetrations-Cluster (Eingang)"=w965) -> ("Pump Concetrations-Cluster (Ausgang)"=w964:T167)  [unwired: 10 in]
                n614 = local write "Pump 1"(w967) -> ()
                n615 = local write "Pump 2"(w964) -> ()
                n616 = local write "MFC0"(w973) -> ()
                n617 = local write "MFC1"(w972) -> ()
                n618 = local write "MFC2"(w971) -> ()
                n619 = local write "MFC3"(w970) -> ()
                n620 = local write "MFC4"(w969) -> ()
                n621 = call "FGV_HovaCAL_Interface_AutoLin_MFC.vi"("Aktion"=enum16{"lesen", "schreiben"}."lesen") -> ("AutoLin MFC out"=w983:u16)  [unwired: 7 in, 3 out]
                n622 = local write "HovaCAL AutoLin MFC"(w983) -> ()
                n623 = call "FGV_HovaCAL_Interface_GetData.vi"("Aktion"=Aktion_FGV_HovaCAL_Interface_GetData."reset after read", "reset index"=0) -> ()  [unwired: 5 in, 5 out]
              }
            }
            n624 = call "Set Values From HovaCAL Output.vi"("error in (no error)"=w947) -> ("error out"=w952:errorcluster, "Cluster.Flow Output Cluster (Ausgang)"=→"Cluster.Flow Output Cluster (Ausgang)" →"Cluster.Flow Output Cluster (Ausgang) 2":cluster{"total flow":dbl}, "Cluster.Pump MassFlow-Cluster"=→"Cluster.Pump MassFlow-Cluster":T171, "Cluster.Pump Concentrations-Cluster"=w935:T172, "Cluster.PumpModeGeneral-Cluster"=→"Cluster.PumpModeGeneral-Cluster" →"Cluster.PumpModeGeneral-Cluster 2":cluster{"running?":bool, "Speed":dbl[]}, "Cluster.Temp Cluster"=→"Cluster.Temp Cluster":T173, "PumpMode-Cluster"=→"HovaCAL SetPumpMode-Cluster out":T163, "MFC Output Array"=w925:T45[])  [unwired: 3 out]
            n625 = call <vilib>:"Clear Errors.vi"("error in (no error)"=w952) -> ()  [unwired: 5 in, 2 out]
            n626 = Index Array(array=w925) -> (element #1=→"MFC Output 0":T45, element #2=→"MFC Output 1":T45, element #3=→"MFC Output 2":T45, element #4=→"MFC Output 3":T45, element #5=→"MFC Output 4":T45)  [unwired: 5 in]
            n627 = Index Array(array=w935) -> (element #1=w929:T174, element #2=w927:T174)  [unwired: 2 in]
            n628 = call "Pump Output in Procent.vi"("Cluster.Pump Concentrations-Cluster"=w929) -> ("Pump Output out"=→"Pump Output 1":T174)  [unwired: 10 in]
            n629 = call "Pump Output in Procent.vi"("Cluster.Pump Concentrations-Cluster"=w927) -> ("Pump Output out"=→"Pump Output 2":T174)  [unwired: 10 in]
          }
          frame "Kalibrierung" {
            n630 = call "FGV Gasteiler.vi"("Aktionen"=Aktionen_FGV_Gasteiler_Daten."lesen") -> ("Gasteiler Type"=w1005:T15, "Anforderung"=w1004:bool)  [unwired: 11 in, 6 out]
            n631 = case shown="True" w1004 {
              tunnel: w1013 -> [_ w1052]
              tunnel: [_ w1053] -> w1012
              tunnel: w1005 -> [_ w1051]
              frame False {
              }
              frame True {
                n632 = case shown="True" w1052 {
                  tunnel: [T4 FALSE ("Gasteiler Spülen") w1056] -> w1053
                  tunnel: w1051 -> [_ w1055]
                  frame False {
                  }
                  frame True {
                    n633 = case shown="0, Standard" w1055 {
                      tunnel: [w1058 w1065] -> w1056
                      frame 0, Default {
                        n634 = call "AK Komm.vi"("Aktionen"=Aktionen_AK_Komm."ASTZ") -> ("Status"=w1057:string)  [unwired: 4 in, 6 out]
                        "Status kalibrieren" <- w1057
                        n635 = Concatenate Strings("Remote", "\n", "Standby") -> (w1059:string)
                        n636 = Equal?(x=w1059, y=w1057) -> (x = y?=w1058:bool)
                      }
                      frame 1 {
                        n637 = call "AK Komm_ALT.vi"("Aktionen_ALT"=Aktionen_AK_Komm_ALT."ASTZ") -> ("Status"=w1064:string)  [unwired: 6 in, 4 out]
                        n638 = local write "Status kalibrieren"(w1064) -> ()
                        n639 = Match Pattern(string=w1064, regular expression="STBY" ("Regulärer Ausdruck")) -> (match substring=w1067:string)  [unwired: 1 in, 3 out]
                        n640 = Empty String/Path?(string/path=w1067) -> (empty?=w1065:bool)
                      }
                    }
                  }
                }
              }
            }
            n641 = property on="Status kalibrieren" class="Str"("Text.Scroll Position"=u32 9999 ("Text.Anzeigeposition")) -> (error out=w1009:errorcluster)  [unwired: 2 in, 1 out]
            n642 = call <vilib>:"Clear Errors.vi"("error in (no error)"=w1009) -> ()  [unwired: 5 in, 2 out]
            n643 = local read "Kalibrier Optionen:"() -> (w1011:enum32{"Gasteiler", "ohne Gasteiler", "PNS"})
            n644 = case shown="\"Gasteiler\", Standard" w1011 {
              frame "Gasteiler", Default {
                w1014 = FALSE
                w1022 = TRUE
                n645 = disable-structure shown="FID==TRUE" {
                  disable-tunnel: w1022 -> [w1028 _]
                  disable-tunnel: [w1027 _] -> w1021
                  disable-tunnel: [w1026 _] -> w1020
                  frame condition #0 {
                    n646 = property on="FID 0 kalibrieren" class="Bool."("Visible"=w1028) -> (error out=w1027:errorcluster)  [unwired: 2 in, 1 out]
                    n647 = property on="FID E kalibrieren" class="Bool."("Visible"=w1028) -> (error out=w1026:errorcluster)  [unwired: 2 in, 1 out]
                  }
                  frame condition #1 (active) {
                  }
                }
                n648 = disable-structure shown="PMA==TRUE" {
                  disable-tunnel: w1022 -> [w1025 _]
                  disable-tunnel: [w1024 _] -> w1019
                  disable-tunnel: [w1023 _] -> w1018
                  frame condition #0 {
                    n649 = property on="PMD 0 kalibrieren" class="Bool."("Visible"=w1025) -> (error out=w1024:errorcluster)  [unwired: 2 in, 1 out]
                    n650 = property on="PMD  E kalibrieren" class="Bool."("Visible"=w1025) -> (error out=w1023:errorcluster)  [unwired: 2 in, 1 out]
                  }
                  frame condition #1 (active) {
                  }
                }
                n651 = property on="FID kalibrieren" class="Bool."("Visible"=w1014) -> (error out=w1016:errorcluster)  [unwired: 2 in, 1 out]
                n652 = property on="PMD kalibrieren" class="Bool."("Visible"=w1014) -> (error out=w1015:errorcluster)  [unwired: 2 in, 1 out]
                n653 = Merge Errors(w1021, w1020, w1019, w1018, w1016, w1015) -> (w1017:errorcluster)
                n654 = call <vilib>:"Clear Errors.vi"("error in (no error)"=w1017) -> ()  [unwired: 5 in, 2 out]
              }
              frame "PNS" {
                w1029 = FALSE
                w1037 = TRUE
                n655 = property on="FID 0 kalibrieren" class="Bool."("Visible"=w1037) -> (error out=w1036:errorcluster)  [unwired: 2 in, 1 out]
                n656 = property on="FID E kalibrieren" class="Bool."("Visible"=w1037) -> (error out=w1035:errorcluster)  [unwired: 2 in, 1 out]
                n657 = property on="PMD 0 kalibrieren" class="Bool."("Visible"=w1037) -> (error out=w1034:errorcluster)  [unwired: 2 in, 1 out]
                n658 = property on="PMD  E kalibrieren" class="Bool."("Visible"=w1037) -> (error out=w1033:errorcluster)  [unwired: 2 in, 1 out]
                n659 = property on="FID kalibrieren" class="Bool."("Visible"=w1029) -> (error out=w1031:errorcluster)  [unwired: 2 in, 1 out]
                n660 = property on="PMD kalibrieren" class="Bool."("Visible"=w1029) -> (error out=w1030:errorcluster)  [unwired: 2 in, 1 out]
                n661 = Merge Errors(w1036, w1035, w1034, w1033, w1031, w1030) -> (w1032:errorcluster)
                n662 = call <vilib>:"Clear Errors.vi"("error in (no error)"=w1032) -> ()  [unwired: 5 in, 2 out]
              }
              frame "ohne Gasteiler" {
                w1041 = TRUE
                w1046 = FALSE
                n663 = disable-structure shown="FID==FALSE, Standard" {
                  disable-tunnel: w1041 -> [w1050 _]
                  disable-tunnel: [w1049 _] -> w1040
                  frame condition #0 {
                    n664 = property on="FID kalibrieren" class="Bool."("Visible"=w1050) -> (error out=w1049:errorcluster)  [unwired: 2 in, 1 out]
                  }
                  frame condition #1 (active) {
                  }
                }
                n665 = disable-structure shown="PMA==FALSE, Standard" {
                  disable-tunnel: w1041 -> [w1048 _]
                  disable-tunnel: [w1047 _] -> w1039
                  frame condition #0 {
                    n666 = property on="PMD kalibrieren" class="Bool."("Visible"=w1048) -> (error out=w1047:errorcluster)  [unwired: 2 in, 1 out]
                  }
                  frame condition #1 (active) {
                  }
                }
                n667 = property on="FID 0 kalibrieren" class="Bool."("Visible"=w1046) -> (error out=w1045:errorcluster)  [unwired: 2 in, 1 out]
                n668 = property on="FID E kalibrieren" class="Bool."("Visible"=w1046) -> (error out=w1038:errorcluster)  [unwired: 2 in, 1 out]
                n669 = property on="PMD 0 kalibrieren" class="Bool."("Visible"=w1046) -> (error out=w1044:errorcluster)  [unwired: 2 in, 1 out]
                n670 = property on="PMD  E kalibrieren" class="Bool."("Visible"=w1046) -> (error out=w1043:errorcluster)  [unwired: 2 in, 1 out]
                n671 = Merge Errors(w1045, w1038, w1044, w1043, w1040, w1039) -> (w1042:errorcluster)
                n672 = call <vilib>:"Clear Errors.vi"("error in (no error)"=w1042) -> ()  [unwired: 5 in, 2 out]
              }
            }
          }
          frame "Daten aufzeichnen" {
            # "#HovaCALMultiMFC #GD_Error_in_Status"
            n673 = local read "Gasnummer Generieren"() -> (w1081:T49)
            n674 = local read "passive Komponente:"() -> (w1076:u16)
            n675 = To Single Precision Float(number=w1083) -> (single precision float=→"Restlaufzeit":sgl)
            n676 = call "Komponentenausgabe HovaCAL fix.vi"("Gasnummer in"=w1081) -> ("Gaskomponente"=w1078:T7)  [unwired: 7 in, 3 out]
            n677 = Equal To 0?(x=w1076) -> (x = 0?=w1080:bool)
            n678 = Decrement(x=w1076) -> (x-1=w1079:u16)
            n679 = Select(t=w1078, s=w1080, f=w1079) -> (s? t:f=w1077:T7)
            n680 = disable-structure shown="Aktiviert" {
              disable-tunnel: w1077 -> [w1108 w1123]
              disable-tunnel: [w1107 w1122] -> w1075
              frame Disabled {
                n681 = call "Polynom Daten speichern.vi"("Aktionen"=Aktionen_Polynom_Daten_speichern."lesen") -> ("Aktiv"=w1119:bool[], "Polynome"=w1120:dbl[][])  [unwired: 5 in, 4 out]
                n682 = Index Array(array=w1120, index (row)=w1108) -> (element=w1107:dbl[])  [unwired: 1 in]
                n683 = Index Array(array=w1119, index=w1108) -> (element=w1118:bool)
                n684 = Select(t=u32 6618880, s=w1118, f=u32 13816530 ("Farbfeld")) -> (s? t:f=w1109:u32)
                n685 = property on="Offset" class="DigWert (strikt)"("NumText.BGColor"=w1109) -> (error out=w1114:errorcluster)  [unwired: 2 in, 1 out]
                n686 = property on="O.1" class="DigWert (strikt)"("NumText.BGColor"=w1109) -> (error out=w1113:errorcluster)  [unwired: 2 in, 1 out]
                n687 = property on="O. 2" class="DigWert (strikt)"("NumText.BGColor"=w1109) -> (error out=w1112:errorcluster)  [unwired: 2 in, 1 out]
                n688 = property on="O. 3" class="DigWert (strikt)"("NumText.BGColor"=w1109) -> (error out=w1111:errorcluster)  [unwired: 2 in, 1 out]
                n689 = property on="O. 4" class="DigWert (strikt)"("NumText.BGColor"=w1109) -> (error out=w1110:errorcluster)  [unwired: 2 in, 1 out]
                n690 = Merge Errors(w1114, w1113, w1112, w1111, w1110) -> (w1115:errorcluster)
                n691 = call <vilib>:"Clear Errors.vi"("error in (no error)"=w1115) -> ()  [unwired: 5 in, 2 out]
              }
              frame Enabled {
                # "#LIN_only_saved_Polynom"
                n692 = call "Polynom Daten speichern.vi"("Aktionen"=Aktionen_Polynom_Daten_speichern."aktiv abfragen", "Komponente"=w1123) -> ("Einzelnes Polynom out"=w1122:dbl[])  [unwired: 4 in, 5 out]
              }
            }
            n693 = call "FGV Gasliste.vi"("Aktionen"=FGV_FT-IR_Gasliste_Aktionen."lesen") -> ("Aktuelle Gasliste gesamt"=w1100:T48[])  [unwired: 8 in, 2 out]
            n694 = call "IstWerte Anzeige.vi"("Gaskomponete"=w1077) -> ("Standardabweichung"=→"Schwankung":sgl, "Messwerte"=→"Istwert":sgl)  [unwired: 7 in, 2 out]
            n695 = Build Array (concatenate)("----", w1100) -> (w1098:T48[])
            n696 = Increment(x=w1077) -> (x+1=w1097:T7)
            n697 = Index Array(array=w1098, index=w1097) -> (element=→"Komponente Daten Gen":T48)
            n698 = Select(t=u32 10812386 ("Farbfeld"), s=w1085, f=u32 13816530 ("Farbfeld")) -> (s? t:f=w1091:u32)
            n699 = Array To Cluster(array=w1075) -> (cluster=→"Polynom":T175)
            n700 = disable-structure shown="Deaktiviert" {
              disable-tunnel: [w1103 w1106] -> w1084
              disable-tunnel: w1077 -> [w1102 w1106]
              frame Disabled {
                # "#WARUM"
                n701 = flat-sequence {
                  tunnel: w1102 -> [w1105]
                  tunnel: [w1105] -> w1103
                  frame #0 {
                    n702 = Wait Until Next ms Multiple(millisecond multiple=u32 500 ("ms")) -> ()  [unwired: 1 out]
                  }
                }
              }
              frame Enabled {
              }
            }
            n703 = property on="Status" class="Str"("Text.BG Color"=w1091) -> (error out=w1090:errorcluster)  [unwired: 2 in, 1 out]
            n704 = case shown="True" w1086 {
              tunnel: w1084 -> [w1126 _]
              tunnel: w1071 -> [w1125 w1132]
              tunnel: [w1125 w1132] -> w1070
              frame True {
                # "Anzeigebit erst löschen\nwenn er in diesem Case\nwar"
                n705 = call "Lin Daten aufarbeiten.vi"("Index (Seite)"=w1126, "Aktionen"=Aktion_Lin_Daten_aufarbeiten."lesen") -> ("Eingabetabelle"=w1130:T54)  [unwired: 15 in, 10 out]
                n706 = call "AusgabeTabelle zusammenbauen.vi"("Eingabetabelle"=w1130) -> ("Eingabetabelle behandelt"=w1128:string[][], "Ausgabetabelle"=w1131:T53)  [unwired: 8 in, 1 out]
                n707 = local write "Ausgabetabelle"(w1131) -> ()
                n708 = local write "Eingabetabelle"(w1128) -> ()
                n709 = call "FGV Daten Abholung uebergeben.vi"("Aktion"=Aktion_FGV_Daten_Abholung_uebergebenctl."Anzeigebit löschen") -> ()  [unwired: 10 in, 5 out]
              }
              frame False {
              }
            }
            n710 = call <vilib>:"Clear Errors.vi"("error in (no error)"=w1090) -> ()  [unwired: 5 in, 2 out]
            n711 = call "GD Errors in Status.vi"("get Test Data"=w1069, "Sprachliste"=w1072, "Status in"=w1070) -> ("Statusout"=→"Status":string)  [unwired: 7 in, 1 out]
          }
          frame "LIN Anpassung" {
            # "#AutorangeSpanfactorsOffsets"
            n712 = call "FGV Gasliste.vi"("Aktionen"=FGV_FT-IR_Gasliste_Aktionen."lesen") -> ("Aktuelle Gasliste gesamt"=w1143:T48[])  [unwired: 8 in, 2 out]
            n713 = Build Array (concatenate)("----", w1143) -> (w1141:T48[])
            n714 = Increment(x=w1135) -> (x+1=w1140:T7)
            n715 = Index Array(array=w1141, index=w1140) -> (element=→"Komponentenanzeige LIN":T48)
            n716 = call "Lin Daten aufarbeiten.vi"("Aktionen"=Aktion_Lin_Daten_aufarbeiten."lesen") -> ("Lin-Polynom"=w1133:T119)  [unwired: 16 in, 10 out]
            n717 = Unbundle By Name(w1133) -> ("Polynomkoeff."=w1134:dbl[], "F_max in % LIN"=w1151:sgl, "F_max gefordert (%)"=w1157:sgl)
            "LIN Max. Error in %:" <- w1151
            n718 = Less?(x=w1151, y=w1157) -> (x < y?=w1156:bool)
            n719 = Select(t=u32 6618880, s=w1156, f=u32 16711680) -> (s? t:f=w1153:u32)
            n720 = Index Array(array=w1134) -> (element=w1150:dbl)  [unwired: 1 in]
            n721 = property on="LIN Max. Error in %:" class="DigWert (strikt)"("NumText.BGColor"=w1153) -> (error out=w1152:errorcluster)  [unwired: 2 in, 1 out]
            n722 = Absolute Value(x=w1150) -> (abs(x)=w1149:dbl)
            n723 = Greater Or Equal?(x=w1149, y=sgl 0.3) -> (x >= y?=w1147:bool)
            n724 = call <vilib>:"Clear Errors.vi"("error in (no error)"=w1152) -> ()  [unwired: 5 in, 2 out]
            n725 = property on="Offset" class="DigWert (strikt)"("Blinking"=w1147) -> (error out=w1146:errorcluster)  [unwired: 2 in, 1 out]
            n726 = call <vilib>:"Clear Errors.vi"("error in (no error)"=w1146) -> ()  [unwired: 5 in, 2 out]
          }
          frame "EPA 1065-307" {
            n727 = call "FGV Gasliste.vi"("Aktionen"=FGV_FT-IR_Gasliste_Aktionen."lesen") -> ("Aktuelle Gasliste gesamt"=w1166:T48[])  [unwired: 8 in, 2 out]
            n728 = Build Array (concatenate)("----", w1166) -> (w1164:T48[])
            n729 = Increment(x=w1161) -> (x+1=w1163:T7)
            n730 = Index Array(array=w1164, index=w1163) -> (element=→"Komponentenanzeige EPA":T48)
          }
          frame "Polynomkoeffizienten" {
            # "#BugFix71"
            n731 = property on="PolynomTabelleEingabe" class="Tbl (strikt)"() -> (error out=w1175:errorcluster, "Index Values"=w1170:T176)  [unwired: 2 in, 1 out]
            n732 = Not Equal?(x=w1171, y=w1170) -> (x != y?=w1174:cluster{"Row":bool, "Column":bool})
            n733 = Cluster To Array(cluster=w1174) -> (array=w1173:bool[])
            n734 = Or Array Elements(Boolean array=w1173) -> (logical OR=w1172:bool)
            n735 = case shown="True" w1172 {
